vi "HGF_FGV_Subset.appendData2Variant.vi"(0 "initData":variant, 2 "index":u32, 3 "length":i32, 5 "error in (no error)":errorcluster) -> (14 "dup initData":variant, 19 "error out":errorcluster)   [LabVIEW 2012, in "HGF_FGV.lvlib" / "HGF_FGV_SubSet.lvclass"]
doc: "Append object initialization data to Variant as attribute."
uses:
  HGF_FGV_SubSet.lvclass
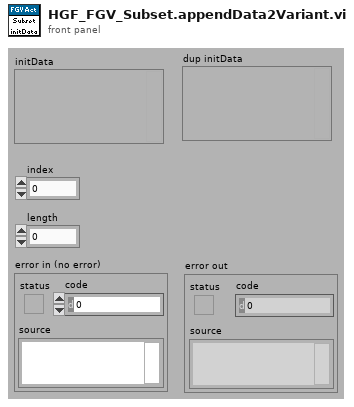
[diagram p1: front panel]
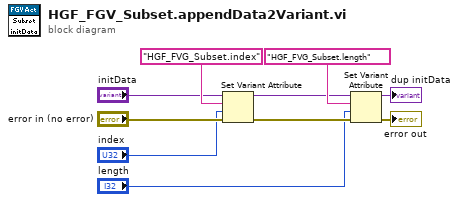
[diagram p0: block diagram]
diagram:
  n1 = Set Variant Attribute(Variant="initData", name="HGF_FVG_Subset.index", value="index", error in="error in (no error)") -> (Variant out=w3:variant, error out=w2:errorcluster)  [unwired: 1 out]
  n2 = Set Variant Attribute(Variant=w3, name="HGF_FVG_Subset.length", value="length", error in=w2) -> (Variant out=→"dup initData":variant, error out=→"error out":errorcluster)  [unwired: 1 out]
